vi "Parse Register Message.vi"(0 "State":string, 1 "Module Name":string, 5 "Args":string) -> (4 "Target":string, 6 "Source":string, 8 "Status":string, 10 "Api":string, 15 "Target Specified?":bool)   [LabVIEW 2017, in "Communicable State Machine.lvlib"]
doc: "### Parse Register Message.vi\n\n-- <b>Controls</b> --\n- <b>state</b>:\n- <b>Module Name </b>:\n- <b>args</b>:\n\n-- <b>Indicators</b> --\n- <b>target</b>:\n- <b>source</b>:\n- <b>status</b>:\n- <b>api</b>:"
uses:
  Communicable State Machine.lvlib
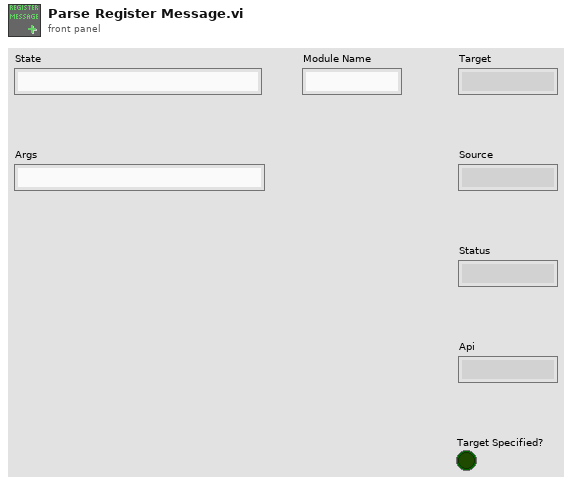
[diagram p1: front panel]
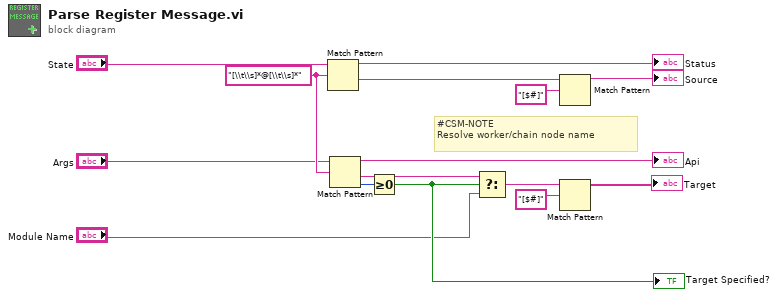
[diagram p0: block diagram]
diagram:
  w12 = "[\\t\\s]*@[\\t\\s]*" ("regular expression")
  # "#CSM-NOTE\nResolve worker/chain node name"
  n1 = Match Pattern(string="State", regular expression=w12) -> (before substring=→"Status":string, after substring=w6:string)  [unwired: 1 in, 2 out]
  n2 = Match Pattern(string="Args", regular expression=w12) -> (before substring=→"Api":string, after substring=w13:string, offset past match=w15:i32)  [unwired: 1 in, 1 out]
  n3 = Greater Or Equal To 0?(x=w15) -> (x >= 0?=w14:bool)
  "Target Specified?" <- w14
  n4 = Select(t=w13, s=w14, f="Module Name") -> (s? t:f=w8:string)
  n5 = Match Pattern(string=w6, regular expression="[$#]") -> (before substring=→"Source":string)  [unwired: 1 in, 3 out]
  n6 = Match Pattern(string=w8, regular expression="[$#]") -> (before substring=→"Target":string)  [unwired: 1 in, 3 out]
